vi "mainUIDisplay.vi"() -> ()   [LabVIEW 2017]
uses:
  <vilib>/Platform/TimedLoop/XDataNode/timing_clust.ctl
  <vilib>/Platform/TimedLoop/XDataNode/nitl_modes.ctl
  <vilib>/Platform/TimedLoop/XDataNode/wakeup.ctl
  opencvSegmentConvertCoordinates-multiFrames.vi
  opencvSelectCandidateNeurons5Planes.vi
  opencvSegment.vi
  opencvSegmentConvertCoordinates-singleFrame.vi
  globalUtilities.vi
  globalDevices.vi
  <vilib>/platform/TimedLoop/XDataNode/XDataNode.xnode
  <vilib>/Analysis/NI_AALBase.lvlib
  <vilib>/Platform/TimedLoop/XDataNode/XDNodeRunTimeDep.lvlib
panel:
  out "objreg":string
  in  "select area":bool
  out "volume direction out":bool
  in  "targetAutoIndex":i32
  in  "targetMode":u16(ring) items=["manual", "auto"]
  in  "save":bool
  out "volumesSaved":i32
  in  "z-profile refresh":bool
  in  "refresh":bool=TRUE
  out "framesNotSaved":i32
  in  "etlLatencyShift":i8
  in  "set etl0 lat shift":bool
  in  "etl1 dpt":dbl
  in  "set etl1 z":bool
  in  "dx":i16
  in  "x0":i16
  in  "dy":i16
  in  "y0":i16
  out "optog etl1 z target\n(in imaging etl0 space)":dbl
  in  "target":bool
  in  "stop":bool
  out "z-profile":cluster{dbl[], dbl[]}[](graph)
  in  "axis":u16(ring) items=["x", "y", "z"]
  in  "GUI refresh time":i64=200
  out "ZX or ZY":u64[][](graph)
  out "XY":u64[][](graph)
  # "DISPLAY BACKEND ACQUISITION\n(run main/backend/mainRecord.vi)"
  # "SETTINGS"
  # "ms"
  # "For the params of the experiment, \nsee main/backend/mainRecord."
  # "This only works if you are running \nthe dyn-reg subVI."
  # "OPTOGENETICS"
  # "(-1: all)"
  # "DIAGNOSTICS"
  # "Z PROFILE"
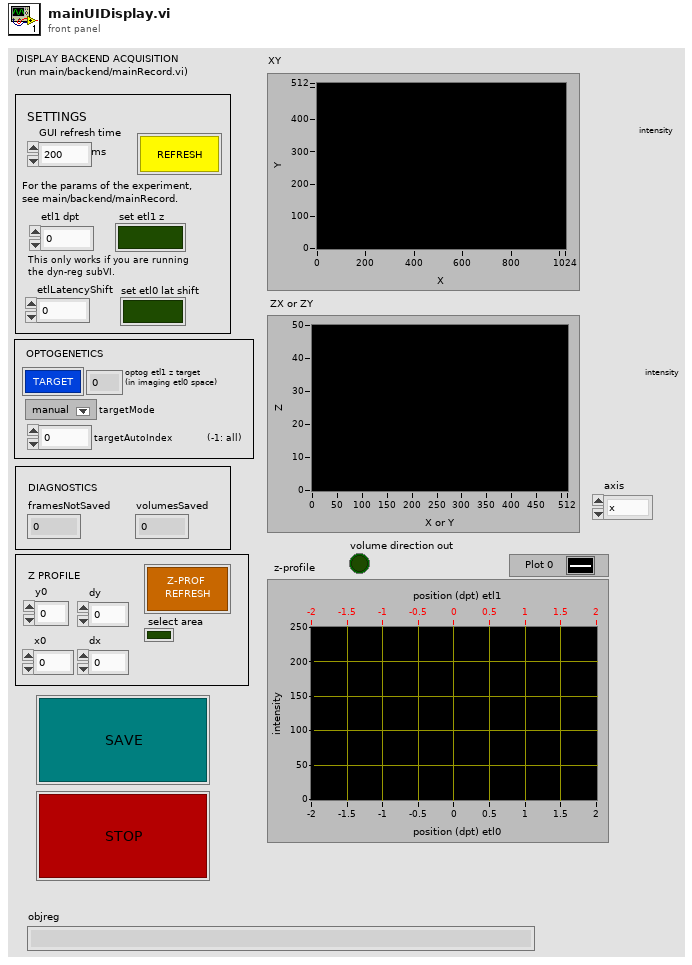
[diagram p1: front panel]
types:
  T1 = typedef "XDNodeRunTimeDep.lvlib/timing_clust.ctl" = cluster{"Expected End [f-1]":u64, "Actual End [f-1]":u64, "Finished Late? [f-1]":bool, "Expected End [i-1]":u64, "Actual End [i-1]":u64, "Finished Late? [i-1]":bool, "Expected Start [i]":u64, "Actual Start [i]":u64, "Expected Start [f]":u64, "Actual Start [f]":u64, "Source Name":string, "Structure Name":string, "Period":i64, "Deadline":i64, "Offset":i64, "Start":i64, "Priority":i32, "Timeout":i32, "Mode":T2, "Wakeup Reason":T3, "Error":errorcluster, "Source Type":string, "Secondary Source Type":string, "Global End Time":u64, "Global Start Time":u64, "Frame Duration":u64, "Iteration Duration":u64, "Assigned CPU":i32, "I/O Scan Engine Mode":u32}
  T2 = typedef "XDNodeRunTimeDep.lvlib/nitl_modes.ctl" = enum32{"No Change", "Process missed periods, maintain original phase", "Discard missed periods, maintain original phase", "Process missed periods, ignore original phase", "Discard missed periods, ignore original phase"}
  T3 = typedef "XDNodeRunTimeDep.lvlib/wakeup.ctl" = enum32{"Normal", "Aborted", "Asynchronous wakeup", "Timing source error", "Timed loop error", "Timeout"}
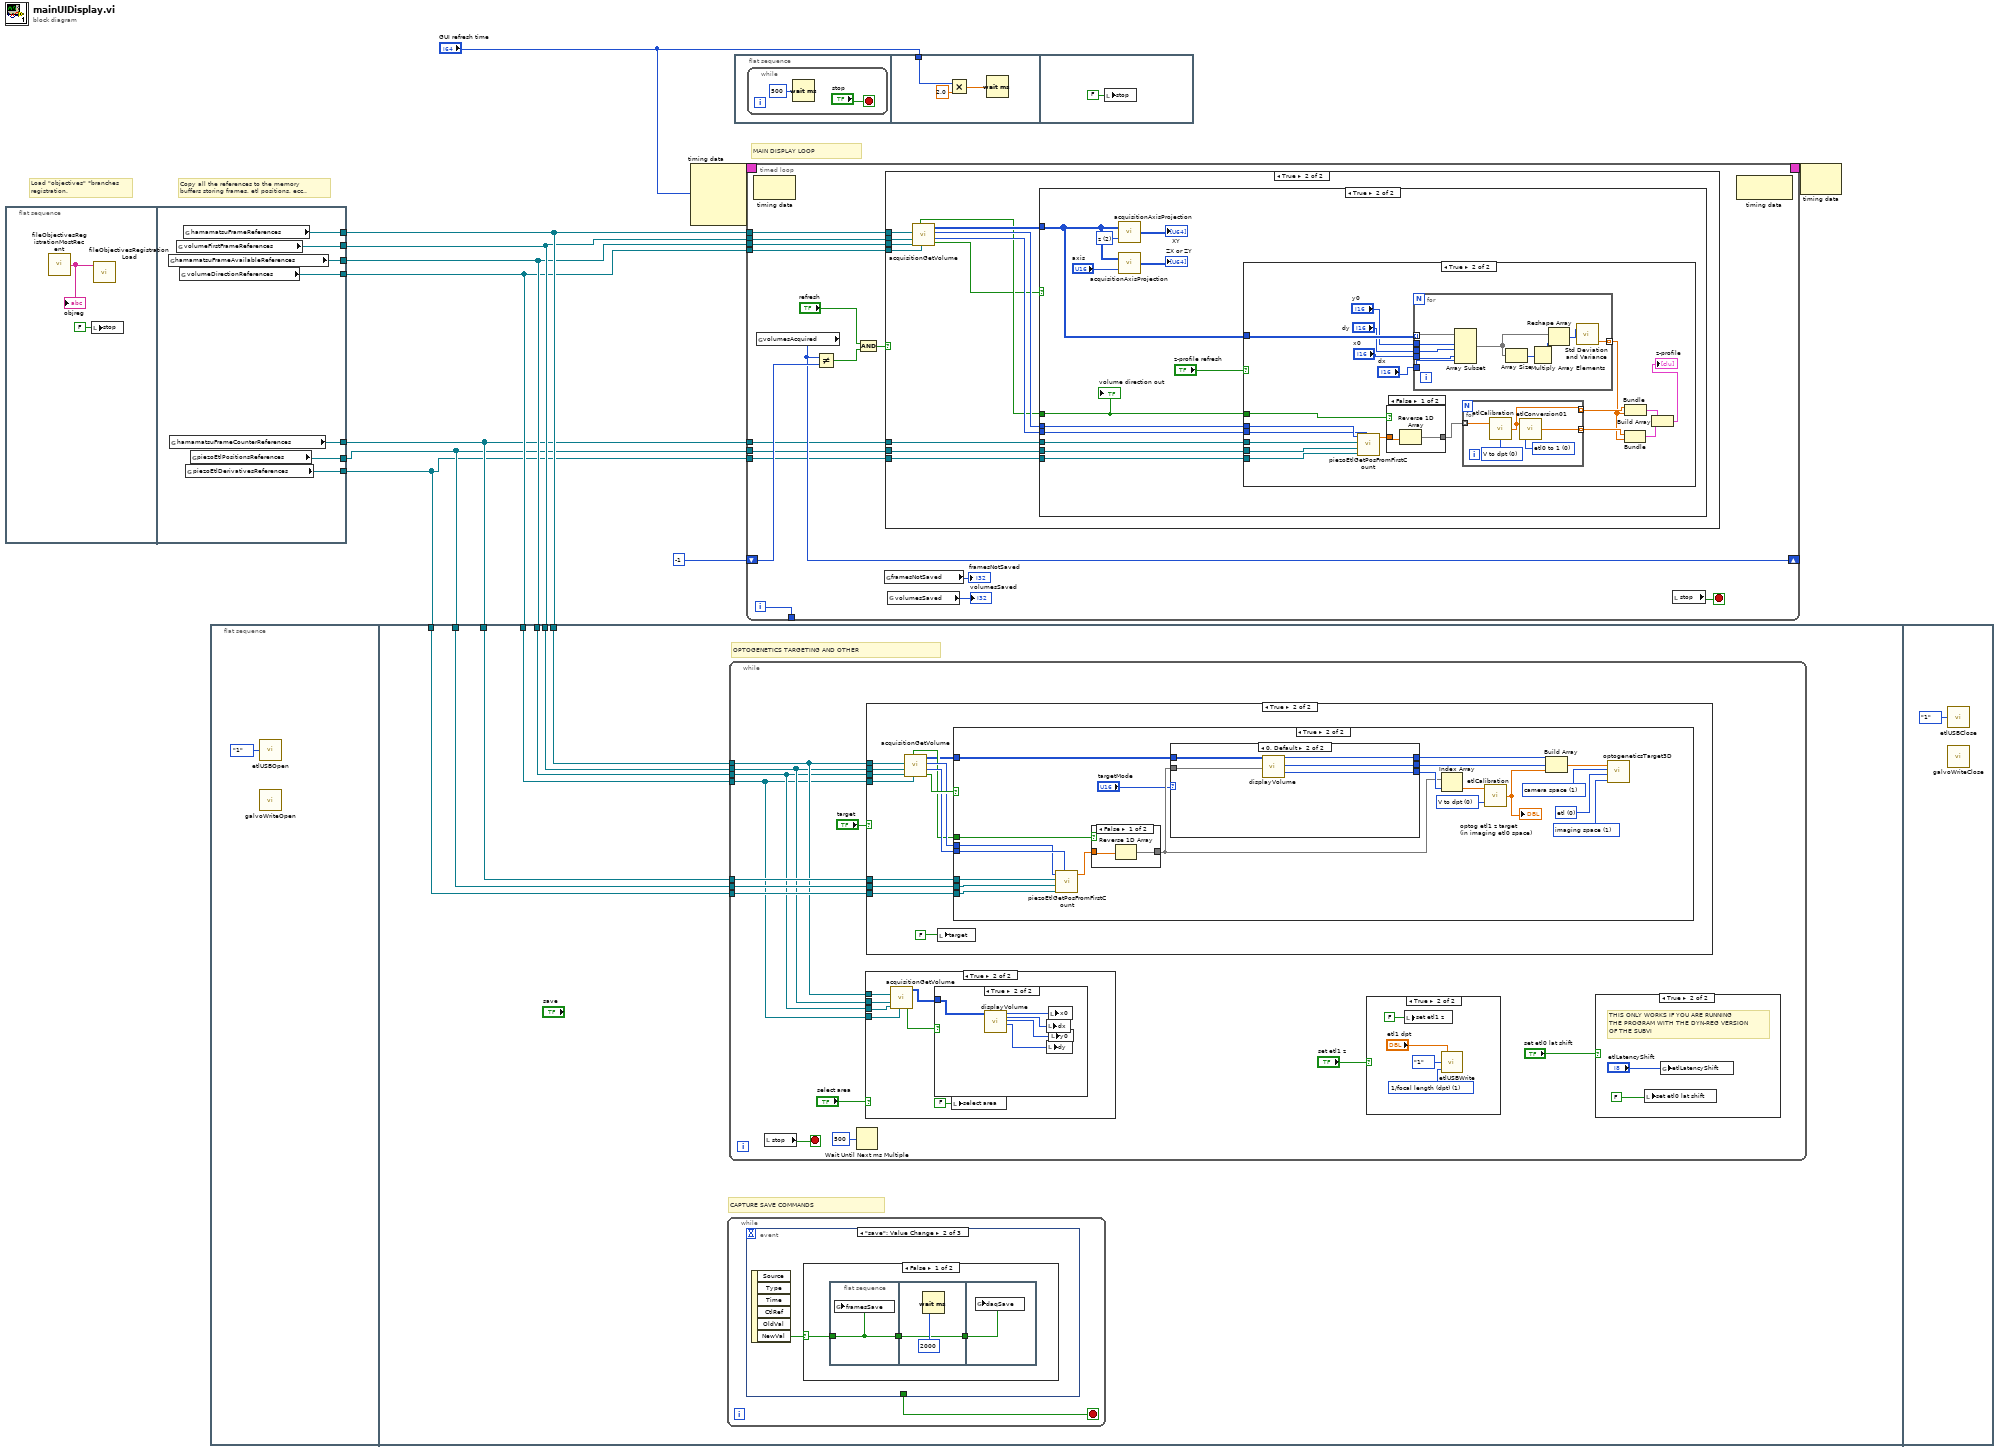
[diagram p0: block diagram]
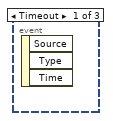
[diagram p6: hidden frame]
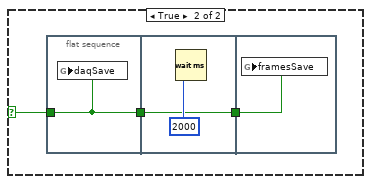
[diagram p7: hidden frame]
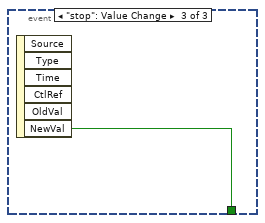
[diagram p8: hidden frame]
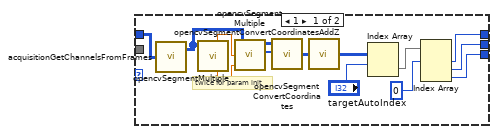
[diagram p15: hidden frame]
diagram:
  # "Copy all the references to the memory\nbuffers storing frames, etl positions, ecc.."
  # "Load \"objectives\" *branches\nregistration."
  # "MAIN DISPLAY LOOP"
  n1 = flat-sequence {
    tunnel: [w20] -> w11
    tunnel: [w19] -> w10
    tunnel: [w18] -> w9
    tunnel: [w17] -> w8
    tunnel: [w16] -> w4
    tunnel: [w15] -> w5
    tunnel: [w14] -> w6
    frame #0 {
      n2 = call "fileObjectivesRegistrationMostRecent.vi"() -> ("f"=w13:string)  [unwired: 1 in]
      "objreg" <- w13
      n3 = local write "stop"(FALSE ("stop")) -> ()
      n4 = call "fileObjectivesRegistrationLoad.vi"("objectiveRegistrationFilePath"=w13) -> ()  [unwired: 3 in, 6 out]
    }
    frame #1 {
      n5 = global read "globalDevices.vi" "hamamatsuFrameAvailableReferences"() -> (w18:refnum<data-value>[])
      n6 = global read "globalDevices.vi" "hamamatsuFrameCounterReferences"() -> (w14:refnum<data-value>[])
      n7 = global read "globalUtilities.vi" "volumeFirstFrameReferences"() -> (w19:refnum<data-value>[])
      n8 = global read "globalUtilities.vi" "volumeDirectionReferences"() -> (w17:refnum<data-value>[])
      n9 = global read "globalDevices.vi" "hamamatsuFrameReferences"() -> (w20:refnum<data-value>[])
      n10 = global read "globalDevices.vi" "piezoEtlDerivativesReferences"() -> (w16:refnum<data-value>[])
      n11 = global read "globalDevices.vi" "piezoEtlPositionsReferences"() -> (w15:refnum<data-value>[])
    }
  }
  n12 = flat-sequence {
    tunnel: w11 -> [w28]
    tunnel: w10 -> [w27]
    tunnel: w9 -> [w26]
    tunnel: w8 -> [w25]
    tunnel: w6 -> [w24]
    tunnel: w5 -> [w23]
    tunnel: w4 -> [w22]
    frame #0 {
      n13 = call "etlUSBOpen.vi"("lens"=enum16{"0", "1"}."1") -> ()  [unwired: 1 in, 1 out]
      n14 = call "galvoWriteOpen.vi"() -> ()  [unwired: 12 in]
    }
    frame #1 {
      # "CAPTURE SAVE COMMANDS"
      # "OPTOGENETICS TARGETING AND OTHER"
      n15 = while {
        stop <- w29 stop-if-true
        n16 = event shown="[1] \"save\": Value Change" {
          selector: _ -> [_ _ _]
          dyn-events: _ -> [_ _ _]
          timeout: _ -> [_ _ _]
          tunnel: [_ _ w45] -> w29
          event Timeout {
            n17 = event-data() -> ()  [unwired: 1 in, 3 out]
          }
          event "save": Value Change {
            n18 = event-data() -> ("NewVal"=w30:bool)  [unwired: 1 in, 5 out]
            n19 = case shown="False" w30 {
              selector: w30 -> [w31 w40]
              frame False {
                n20 = flat-sequence {
                  tunnel: w31 -> [w34]
                  tunnel: [w34] -> w33
                  tunnel: [w35] -> w32
                  tunnel: w33 -> [w35]
                  tunnel: w32 -> [w37]
                  frame #0 {
                    n21 = global write "globalUtilities.vi" "framesSave"(w34) -> ()
                  }
                  frame #1 {
                    n22 = Wait (ms)(milliseconds to wait=u32 2000) -> ()  [unwired: 1 out]
                  }
                  frame #2 {
                    n23 = global write "globalUtilities.vi" "daqSave"(w37) -> ()
                  }
                }
              }
              frame True {
                n24 = flat-sequence {
                  tunnel: w40 -> [w41]
                  tunnel: [w41] -> w38
                  tunnel: [w42] -> w39
                  tunnel: w38 -> [w42]
                  tunnel: w39 -> [w44]
                  frame #0 {
                    n25 = global write "globalUtilities.vi" "daqSave"(w41) -> ()
                  }
                  frame #1 {
                    n26 = Wait (ms)(milliseconds to wait=u32 2000) -> ()  [unwired: 1 out]
                  }
                  frame #2 {
                    n27 = global write "globalUtilities.vi" "framesSave"(w44) -> ()
                  }
                }
              }
            }
          }
          event "stop": Value Change {
            n28 = event-data() -> ("NewVal"=w45:bool)  [unwired: 1 in, 5 out]
          }
        }
      }
      n29 = while {
        tunnel: w28 -> [w50]
        tunnel: w27 -> [w49]
        tunnel: w26 -> [w48]
        tunnel: w25 -> [w47]
        tunnel: w24 -> [w54]
        tunnel: w23 -> [w53]
        tunnel: w22 -> [w52]
        stop <- w57 stop-if-true
        n30 = local read "stop"() -> (w57:bool)
        n31 = Wait Until Next ms Multiple(millisecond multiple=u32 500) -> ()  [unwired: 1 out]
        n32 = case shown="True" "select area" {
          tunnel: w50 -> [_ w65]
          tunnel: w49 -> [_ w64]
          tunnel: w48 -> [_ w63]
          tunnel: w47 -> [_ w62]
          frame False {
          }
          frame True {
            n33 = call "acquisitionGetVolume.vi"("volumeDirectionReferences"=w62, "hamamatsuFrameAvailableReferences"=w63, "volumeFirstFrameReferences"=w64, "hamamatsuFrameReferences"=w65) -> ("success"=w60:bool, "volume out"=w61:u16[][][])  [unwired: 1 in, 3 out]
            n34 = case shown="True" w60 {
              tunnel: w61 -> [_ w70]
              frame False {
              }
              frame True {
                n35 = call "displayVolume.vi"("frames"=w70) -> ("X0out"=w69:i32, "deltaXout"=w68:i32, "Y0out"=w67:i32, "deltaYout"=w66:i32)  [unwired: 13 in, 2 out]
                n36 = local write "dx"(w68) -> ()
                n37 = local write "dy"(w66) -> ()
                n38 = local write "x0"(w69) -> ()
                n39 = local write "y0"(w67) -> ()
              }
            }
            n40 = local write "select area"(FALSE ("select area")) -> ()
          }
        }
        n41 = case shown="True" "target" {
          tunnel: w50 -> [_ w89]
          tunnel: w49 -> [_ w88]
          tunnel: w48 -> [_ w87]
          tunnel: w47 -> [_ w86]
          tunnel: w54 -> [_ w79]
          tunnel: w53 -> [_ w78]
          tunnel: w52 -> [_ w77]
          frame False {
          }
          frame True {
            n42 = call "acquisitionGetVolume.vi"("volumeDirectionReferences"=w86, "hamamatsuFrameAvailableReferences"=w87, "volumeFirstFrameReferences"=w88, "hamamatsuFrameReferences"=w89) -> ("success"=w85:bool, "numberOfFrames"=w83:u32, "absoluteCountFirstFrame"=w84:u32, "volume out"=w81:u16[][][], "volume direction out"=w82:bool)  [unwired: 1 in]
            n43 = local write "target"(FALSE) -> ()
            n44 = case shown="True" w85 {
              tunnel: w84 -> [_ w92]
              tunnel: w83 -> [_ w93]
              tunnel: w82 -> [_ w109]
              tunnel: w81 -> [_ w108]
              tunnel: w79 -> [_ w96]
              tunnel: w78 -> [_ w95]
              tunnel: w77 -> [_ w94]
              frame False {
              }
              frame True {
                w99 = u16 0 items=["V to dpt", "dpt to V"] ("mode")
                w102 = u16 1 items=["optogenetics space", "imaging space"] ("z mode")
                w103 = u16 0 items=["etl", "piezo"] ("z device")
                w104 = u16 1 items=["galvo space", "camera space"] ("xy mode")
                n45 = call "piezoEtlGetPosFromFirstCount.vi"("firstFrameCount"=w92, "hamamatsuFrameCounterReferences"=w96, "piezoEtlPositionsReferences"=w95, "piezoEtlDerivativesReferences"=w94, "nFrames"=w93) -> ("piezoEtlPositions"=w91:dbl[])  [unwired: 2 out]
                n46 = case shown="False" w109 {
                  tunnel: w91 -> [w130 w131]
                  tunnel: [w129 w131] -> w97
                  frame False {
                    n47 = Reverse 1D Array(array=w130) -> (reversed array=w129:dbl[])
                  }
                  frame True {
                  }
                }
                n48 = case shown="0, Default" "targetMode" {
                  tunnel: w108 -> [w118 w128]
                  tunnel: [w112 w125] -> w107
                  tunnel: [w111 w124] -> w106
                  tunnel: [w110 w127] -> w101
                  tunnel: w97 -> [_ w126]
                  frame 1 {
                    # "twice for param init"
                    n49 = call "acquisitionGetChannelsFromFrames.vi"("frameIn"=w118) -> ("Red"=w121:u16[][][])  [unwired: 1 out]
                    n50 = call "opencvSegmentMultiple.vi"("ImgIn"=w121) -> ("maxY"=w119:dbl, "maxX"=w120:dbl)  [unwired: 2 in, 4 out]
                    n51 = call "opencvSegmentMultiple.vi"("maxYInStack"=w119, "maxXInStack"=w120, "ImgIn"=w121) -> ("NeuronN[frame]"=w123:u16[], "NeuronXY[frame]"=w122:u16[][])  [unwired: 4 out]
                    n52 = call-poly "opencvSegmentConvertCoordinates.vi"("NeuronN"=w123, "NeuronXY"=w122) -> ("XY"=w117:u16[][][])  [unwired: 1 in]
                    n53 = call "opencvSegmentConvertCoordinatesAddZ.vi"("XY"=w117) -> ("XYZ"=w116:i32[][])
                    n54 = Index Array(array=w116, index (row)="targetAutoIndex") -> (element=w114:i32[])  [unwired: 1 in]
                    n55 = Index Array(array=w114, index #1=0 ("index")) -> (element #1=w112:i32, element #2=w111:i32, element #3=w110:i32)  [unwired: 2 in]
                  }
                  frame 0, Default {
                    n56 = call "displayVolume.vi"("frames"=w128, "z"=w126) -> ("X0out"=w125:i32, "Y0out"=w124:i32, "zout (plane index)"=w127:i32)  [unwired: 12 in, 3 out]
                  }
                }
                n57 = Index Array(array=w97, index=w101) -> (element=w100:dbl)
                n58 = call "etlCalibration.vi"("mode"=w99, "in"=w100) -> ("out"=w98:dbl)
                "optog etl1 z target\n(in imaging etl0 space)" <- w98
                n59 = Build Array(w107, w106, w98) -> (w105:dbl[])
                n60 = call "optogeneticsTarget3D.vi"("z mode"=w102, "z device"=w103, "xy mode"=w104, "xyz"=w105) -> ()  [unwired: 1 in]
              }
            }
          }
        }
        n61 = case shown="True" "set etl1 z" {
          frame False {
          }
          frame True {
            w75 = u16 1 items=["position (um)", "1/focal length (dpt)"] ("mode")
            n62 = local write "set etl1 z"(FALSE ("select area")) -> ()
            n63 = call "etlUSBWrite.vi"("mode"=w75, "lens"=enum16{"0", "1"}."1", "input"="etl1 dpt") -> ()  [unwired: 1 in]
          }
        }
        n64 = case shown="True" "set etl0 lat shift" {
          frame False {
          }
          frame True {
            # "THIS ONLY WORKS IF YOU ARE RUNNING\nTHE PROGRAM WITH THE DYN-REG VERSION\nOF THE SUBVI"
            n65 = local write "set etl0 lat shift"(FALSE ("set lat shift")) -> ()
            n66 = global write "globalDevices.vi" "etlLatencyShift"("etlLatencyShift") -> ()
          }
        }
      }
    }
    frame #2 {
      n67 = call "etlUSBClose.vi"("lens"=enum16{"0", "1"}."1") -> ()  [unwired: 1 in]
      n68 = call "galvoWriteClose.vi"() -> ()  [unwired: 12 in]
    }
  }
  n69 = node-c288("GUI refresh time") -> (w3:T1)  [unwired: 3 in]
  n70 = flat-sequence {
    tunnel: "GUI refresh time" -> [w137]
    frame #0 {
      n71 = while {
        stop <- "stop" stop-if-true
        n72 = Wait (ms)(milliseconds to wait=u32 500) -> ()  [unwired: 1 out]
      }
    }
    frame #1 {
      n73 = Multiply(x=w137, y=2.0) -> (x*y=w135:dbl)
      n74 = Wait (ms)(milliseconds to wait=w135) -> ()  [unwired: 1 out]
    }
    frame #2 {
      n75 = local write "stop"(FALSE ("stop")) -> ()
    }
  }
  n76 = timed-loop {
    tunnel: w11 -> [w154]
    tunnel: w10 -> [w153]
    tunnel: w9 -> [w152]
    tunnel: w8 -> [w151]
    shift-right: [w148] -> _
    shift-left: -1 -> [w149]
    tunnel: w4 -> [w143]
    tunnel: w5 -> [w142]
    tunnel: w6 -> [w141]
    tunnel: [w140] -> _
    timing: w3 -> [_]
    timing-out: [_] -> w2
    i -> [w140]
    stop <- w150 stop-if-true
    n77 = node-c288() -> ()  [unwired: 1 in, 1 out]
    n78 = global read "globalUtilities.vi" "volumesAcquired"() -> (w148:i32)
    n79 = Not Equal?(x=w148, y=w149) -> (x != y?=w139:bool)
    n80 = And(x="refresh", y=w139) -> (x .and. y?=w146:bool)
    n81 = global read "globalUtilities.vi" "framesNotSaved"() -> (→"framesNotSaved":i32)
    n82 = case shown="True" w146 {
      tunnel: w154 -> [_ w168]
      tunnel: w153 -> [_ w167]
      tunnel: w152 -> [_ w166]
      tunnel: w151 -> [_ w165]
      tunnel: w143 -> [_ w159]
      tunnel: w142 -> [_ w158]
      tunnel: w141 -> [_ w157]
      frame False {
      }
      frame True {
        n83 = call "acquisitionGetVolume.vi"("volumeDirectionReferences"=w165, "hamamatsuFrameAvailableReferences"=w166, "volumeFirstFrameReferences"=w167, "hamamatsuFrameReferences"=w168) -> ("success"=w160:bool, "numberOfFrames"=w162:u32, "absoluteCountFirstFrame"=w163:u32, "volume out"=w164:u16[][][], "volume direction out"=w161:bool)  [unwired: 1 in]
        n84 = case shown="True" w160 {
          tunnel: w164 -> [_ w175]
          tunnel: w163 -> [_ w178]
          tunnel: w162 -> [_ w177]
          tunnel: w161 -> [_ w176]
          tunnel: w159 -> [_ w173]
          tunnel: w158 -> [_ w172]
          tunnel: w157 -> [_ w171]
          frame False {
          }
          frame True {
            w180 = u16 2 items=["x", "y", "z"] ("axis (z)")
            n85 = call "acquisitionAxisProjection.vi"("axis (z)"=w180, "z stack"=w175) -> ("projected img"=→"XY":u64[][])
            n86 = call "acquisitionAxisProjection.vi"("axis (z)"="axis", "z stack"=w175) -> ("projected img"=→"ZX or ZY":u64[][])
            n87 = case shown="True" "z-profile refresh" {
              tunnel: w178 -> [_ w190]
              tunnel: w177 -> [_ w189]
              tunnel: w176 -> [_ w199]
              tunnel: w175 -> [_ w198]
              tunnel: w173 -> [_ w191]
              tunnel: w172 -> [_ w192]
              tunnel: w171 -> [_ w193]
              frame False {
              }
              frame True {
                n88 = call "piezoEtlGetPosFromFirstCount.vi"("firstFrameCount"=w190, "hamamatsuFrameCounterReferences"=w193, "piezoEtlPositionsReferences"=w192, "piezoEtlDerivativesReferences"=w191, "nFrames"=w189) -> ("piezoEtlPositions"=w188:dbl[])  [unwired: 2 out]
                n89 = case shown="False" w199 {
                  tunnel: w188 -> [w206 w207]
                  tunnel: [w205 w207] -> w187
                  frame False {
                    n90 = Reverse 1D Array(array=w206) -> (reversed array=w205:dbl[])
                  }
                  frame True {
                  }
                }
                n91 = for {
                  tunnel: w198 -> [w214] mode=indexing
                  tunnel: "y0" -> [w212]
                  tunnel: "dy" -> [w211]
                  tunnel: "x0" -> [w210]
                  tunnel: "dx" -> [w209]
                  tunnel: [w208] -> w184 mode=indexing
                  n92 = Array Subset(array=w214, index (row)=w212, length (row)=w211, index (col)=w210, length (col)=w209) -> (w213:u16[][])
                  n93 = Array Size(array=w213) -> (size(s)=w217:i32[])
                  n94 = Multiply Array Elements(1:w217) -> (0:w216:i32)
                  n95 = Reshape Array(w213, w216) -> (w215:u16[])
                  n96 = call <vilib>:"Std Deviation and Variance.vi"("X"=w215) -> ("variance"=w208:dbl)  [unwired: 1 in, 2 out]
                }
                n97 = for {
                  tunnel: w187 -> [w204] mode=indexing
                  tunnel: [w201] -> w185 mode=indexing
                  tunnel: [w200] -> w186 mode=indexing
                  w202 = u16 0 items=["V to dpt", "dpt to V"] ("mode")
                  w203 = u16 0 items=["etl0 to 1", "etl1 to 0"] ("mode")
                  n98 = call "etlCalibration.vi"("mode"=w202, "in"=w204) -> ("out"=w200:dbl)
                  n99 = call "etlConversion01.vi"("mode"=w203, "in"=w200) -> ("out"=w201:dbl)
                }
                n100 = Bundle(w185, w184) -> (w182:cluster{dbl[], dbl[]})  [unwired: 1 in]
                n101 = Bundle(w186, w184) -> (w183:cluster{dbl[], dbl[]})  [unwired: 1 in]
                n102 = Build Array(w183, w182) -> (→"z-profile":cluster{dbl[], dbl[]}[])
              }
            }
            "volume direction out" <- w176
          }
        }
      }
    }
    n103 = global read "globalUtilities.vi" "volumesSaved"() -> (→"volumesSaved":i32)
    n104 = local read "stop"() -> (w150:bool)
    n105 = node-c288() -> ()  [unwired: 1 in, 1 out]
  }
  n106 = node-c288(w2) -> ()  [unwired: 1 out]
